vi "Set Up Dialog - Thermistor.vi"() -> ()   [LabVIEW 2012]
panel:
  in  "Done":bool
  # "iWorx - Thermistor - Set Up"
  # "Set Up Instructions"
  # "1. Connect the IX-MYDAQ adaptor board to the NI myDAQ\n\n2. Connect the NI myDAQ to your PC using a USB cable.\n\n3. Connect the TMN-100 to the IX-MYDAQ.\n\n4. Prepare 2 water baths, one at 30oC and the other at 40oC. \n\n5. Put the TMN-100 in the 30oC bath first. Once the trace settles click Set for SP1.\n\n6. Put the TMN-100 in the 40oC bath. Once the trace settles click Set for SP2."
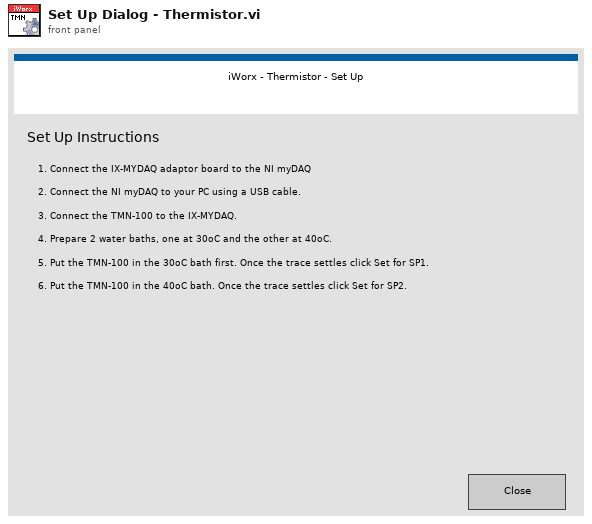
[diagram p1: front panel]
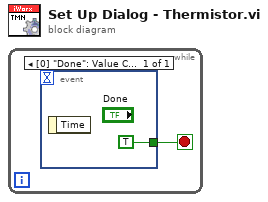
[diagram p0: block diagram]
diagram:
  n1 = while {
    stop <- w1 stop-if-true
    n2 = event shown="[0] \"Done\": Value Change;  Panel Close" {
      selector: _ -> [_]
      dyn-events: _ -> [_]
      timeout: _ -> [_]
      tunnel: [TRUE] -> w1
      event "Done": Value Change; Panel Close {
        n3 = event-data() -> ()  [unwired: 1 in, 1 out]
      }
    }
  }
